vi "GameOver.vi"(1 "背景":dbl[][](array[numeric]), 2 "方块":dbl[][](array[numeric]), 3 "point":cluster{"x":i16, "y":i16} caption="位置") -> (0 "输出":bool)   [LabVIEW 2016]
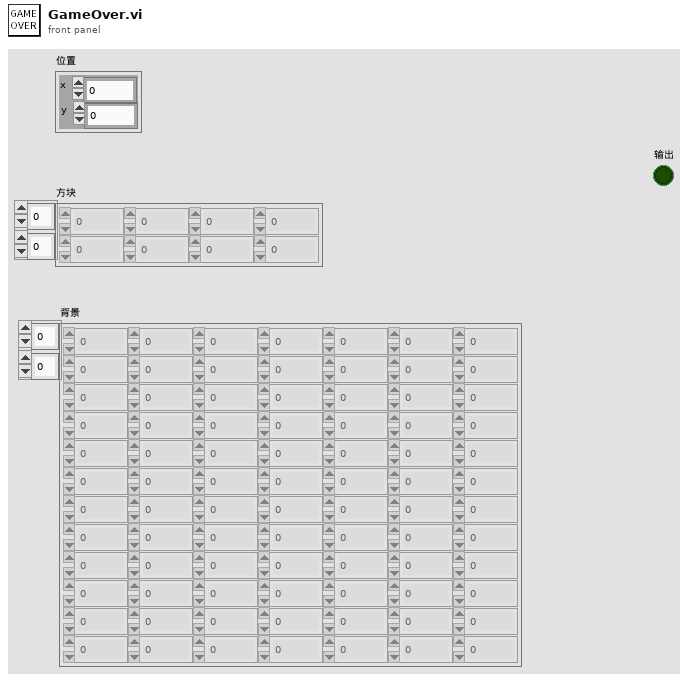
[diagram p1: front panel]
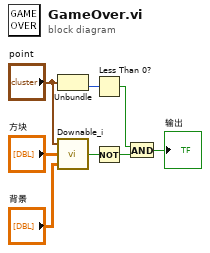
[diagram p0: block diagram]
diagram:
  n1 = Unbundle("point") -> ("y"=w5:i16)  [unwired: 1 out]
  n2 = call "Downable_i.vi"("背景"="背景", "方块"="方块", "point"="point") -> ("输出"=w2:bool)
  n3 = Less Than 0?(x=w5) -> (x < 0?=w4:bool)
  n4 = Not(x=w2) -> (.not. x?=w1:bool)
  n5 = And(x=w4, y=w1) -> (x .and. y?=→"输出":bool)
